vi "MD - Read motion done status.vi"(8 "error in":errorcluster, 10 "Axis":i8=1 min=1 max=6 step=1, 11 "Address / Port":i16=1 min=1 max=31 step=1) -> (0 "error out":errorcluster, 1 "Done":bool, 2 "Axis dup":i8=1 min=1 max=6 step=1, 3 "Address / Port dup":i16=1 min=1 max=31 step=1)   [LabVIEW 2014]
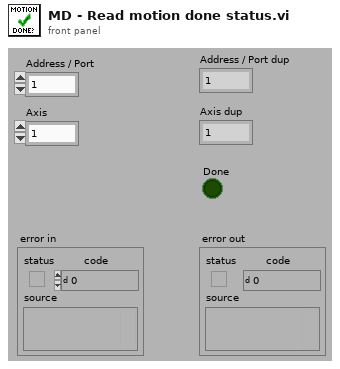
[diagram p1: front panel]
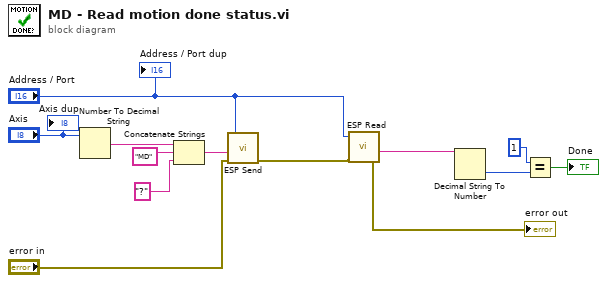
[diagram p0: block diagram]
diagram:
  n1 = Number To Decimal String(number="Axis") -> (decimal integer string=w12:string)  [unwired: 1 in]
  n2 = Concatenate Strings(w12, "MD" ("Substring"), "?" ("Substring")) -> (w10:string)
  n3 = call "ESP Send.vi"("error in"="error in", "Command String"=w10, "Address / Port"="Address / Port") -> ("error out"=w6:errorcluster)  [unwired: 3 in, 1 out]
  n4 = call "ESP Read.vi"("error in"=w6, "Address / Port"="Address / Port") -> ("error out"=→"error out":errorcluster, "Response String"=w4:string)  [unwired: 3 in, 1 out]
  n5 = Decimal String To Number(string=w4) -> (number=w2:i32)  [unwired: 2 in, 1 out]
  n6 = Equal?(x=1 ("y"), y=w2) -> (x = y?=→"Done":bool)
  "Address / Port dup" <- "Address / Port"
  "Axis dup" <- "Axis"
